vi "KB-Sub1-DealWith All Picture.vi"(6 "Color Select":string(combo)="白色", 7 "error in":errorcluster, 8 "Row Select":string(combo)="Item1", 9 "相机分辨率":string, 10 "参数":string[](array[string]), 11 "Image  In":T1(plugin-control)) -> (0 "error out":errorcluster, 1 "结果":string[](array[string]), 2 "数组":sgl[](array[numeric]), 3 "Image Out":T1)   [LabVIEW 2015]
uses:
  <vilib>/vision/Image Controls.llb/IMAQ Image.ctl
panel:
  out "x/y":dbl
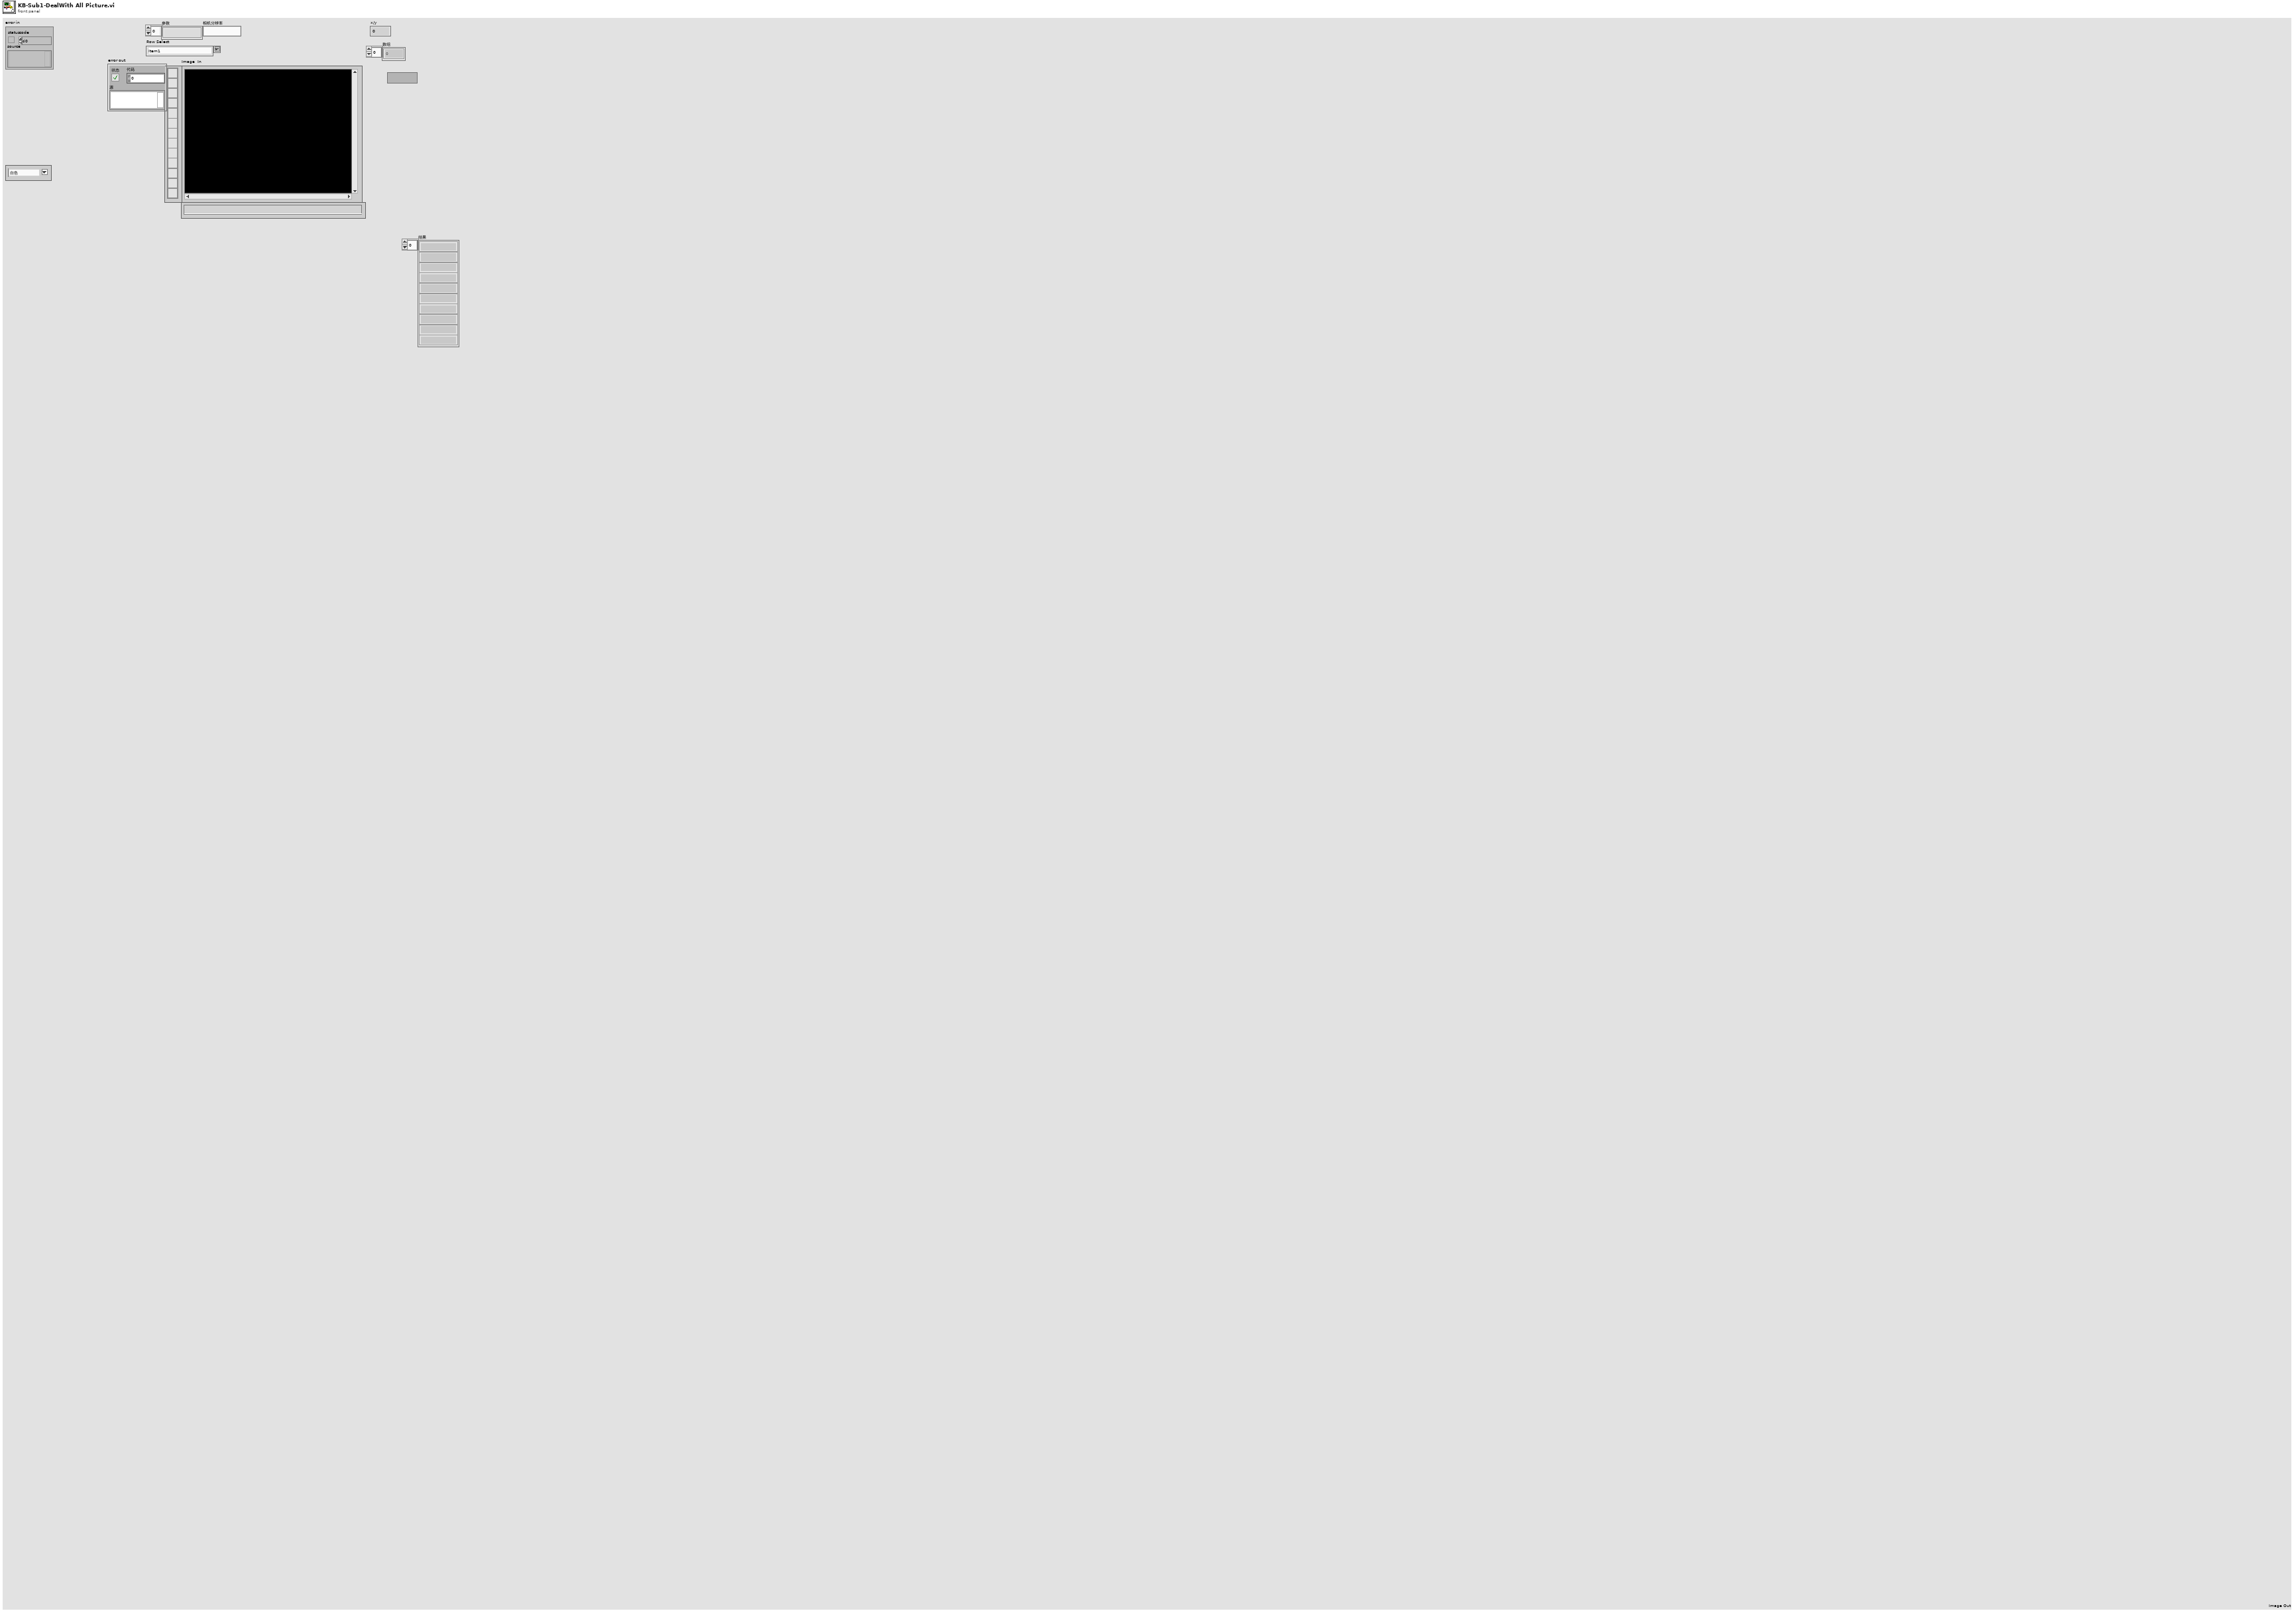
[diagram p1: front panel]
types:
  T1 = typedef "IMAQ Image.ctl" = refnum<image>
  T2 = typedef "ROI Descriptor" = cluster{"Global Rectangle":i32[], "Contours":cluster{"ID":enum32{"External", "Internal"}, "Type":u32, "Coordinates":i32[]}[]}
  T3 = typedef "Edge Options.ctl" = cluster{"Edge Polarity":T4, "Kernel Size":u32, "Width":u32, "Minimum Edge Strength":sgl, "Interpolation Type":enum32{"Zero Order", "Bilinear", "Quadratic", "Cubic", "Bilinear Fixed"}, "Data Processing Method":enum32{"Average", "Median"}}
  T4 = typedef "Edge Polarity.ctl" = u32
  T5 = cluster{"Search  Direction":u32, "Edge Options":T3, "Show Search Area":bool, "Show Search Lines":bool, "Show Edges Found":bool, "Show Result":bool, "Search Area Color":u32, "Search Lines Color":u32, "Edge Locations Color":u32, "Result Color":u32, "Overlay Group Name":string}
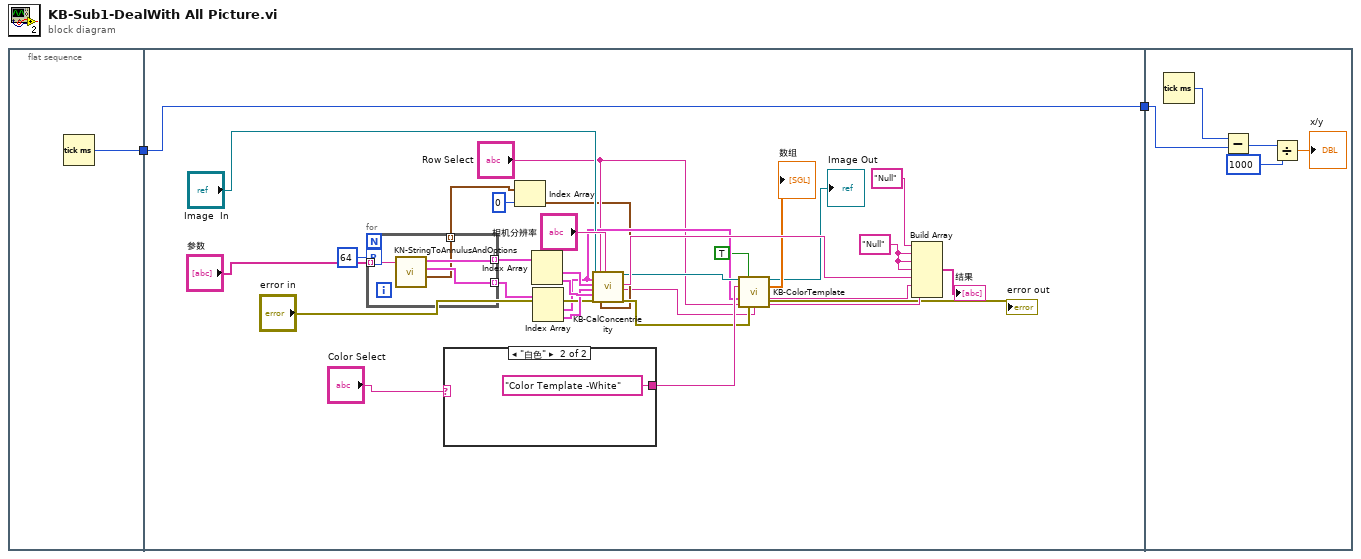
[diagram p0: block diagram]
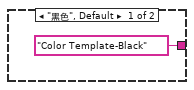
[diagram p2: hidden frame]
diagram:
  n1 = flat-sequence {
    tunnel: [w3] -> w1
    tunnel: [w9] -> w2
    tunnel: w1 -> [w9]
    tunnel: w2 -> [w44]
    frame #0 {
      n2 = Tick Count (ms)() -> (millisecond timer value=w3:u32)
    }
    frame #1 {
      w21 = "Null" ("元素")
      n3 = for {
        tunnel: "参数" -> [w40] mode=indexing
        tunnel: [w39] -> w34 mode=indexing
        tunnel: [w38] -> w33 mode=indexing
        workers-P: 64 -> [_]
        tunnel: [w37] -> w7 mode=indexing
        n4 = call "KN-StringToAnnulusAndOptions.vi"("String"=w40) -> ("Range (Threshold 1)"=w37:cluster{"Lower value":sgl, "Upper value":sgl}, "ROI Descriptor"=w38:T2, "Option All"=w39:T5)  [unwired: 5 in, 3 out]
      }
      n5 = case shown="\"白色\"" "Color Select" {
        tunnel: ["Color Template-Black" ("名称或相对路径") "Color Template -White" ("名称或相对路径")] -> w19
        frame "黑色", Default {
        }
        frame "白色" {
        }
      }
      n6 = Index Array(array=w7, index=0 ("索引")) -> (element=w6:cluster{"Lower value":sgl, "Upper value":sgl})
      n7 = Index Array(array=w34) -> (element #1=w32:T5, element #2=w31:T5)  [unwired: 2 in]
      n8 = Index Array(array=w33) -> (element #1=w11:T2, element #2=w30:T2)  [unwired: 2 in]
      n9 = call "KB-CalConcentrieity.vi"("Image  In"="Image  In", "ROI Descriptor (Otter-Find Circular Edge)"=w11, "Options (Otter-Find Circular Edge)"=w32, "ROI Descriptor (Inner Find Circular Edge 2)"=w30, "Options (Inner Find Circular Edge 2)"=w31, "error in"="error in", "Row Select"="Row Select", "Range (Threshold 1)"=w6, "相机分辨率"="相机分辨率") -> ("Image  Out"=w16:T1, "Concentrieity"=w29:string, "color"=w4:string, "error out"=w14:errorcluster)  [unwired: 5 in, 2 out]
      n10 = call "KB-ColorTemplate.vi"("Image In"=w16, "布尔"=TRUE, "名称或相对路径"=w19, "ROI Descriptor (Color Pattern Matching 1)"=w11, "Row Select"="Row Select", "error in"=w14, "Color"=w4) -> ("Image Out"=→"Image Out":T1, "Score Array"=→"数组":sgl[], "颜色"=w24:string, "error out"=→"error out":errorcluster, "是否漏装"=w23:string)  [unwired: 4 in]
      n11 = Build Array("Null" ("元素"), w21, w21, w21, w29, w24, w23) -> (→"结果":string[])
    }
    frame #2 {
      n12 = Tick Count (ms)() -> (millisecond timer value=w45:u32)
      n13 = Subtract(x=w45, y=w44) -> (x-y=w43:u32)
      n14 = Divide(x=w43, y=u32 1000) -> (x/y=→"x/y":dbl)
    }
  }
